vi "Add Measurement.vi"(8 "error in (no error)":errorcluster, 10 "Measurement":refnum<class "TestManagerMsg.Measurement.lvclass">, 11 "TestManagerMsg.Assertion in":refnum<class "TestManagerMsg.Assertion.lvclass">) -> (0 "error out":errorcluster, 1 "Created/Updated":bool, 3 "TestManagerMsg.Assertion out":refnum<class "TestManagerMsg.Assertion.lvclass">)   [LabVIEW 2013, in "Caraya.lvlib" / "TestManagerMsg.Assertion.lvclass"]
uses:
  TestManagerMsg.Assertion.lvclass
  Test Manager Message Measurement/TestManagerMsg.Measurement.lvclass
  TestManagerMsg.Assertion.lvclass/TestManagerMsg.Assertion.ctl
  Test Manager Message/TestManagerMsg.lvclass/TestManagerMsg.ctl
  Test Manager Message/TestManagerMsg.lvclass
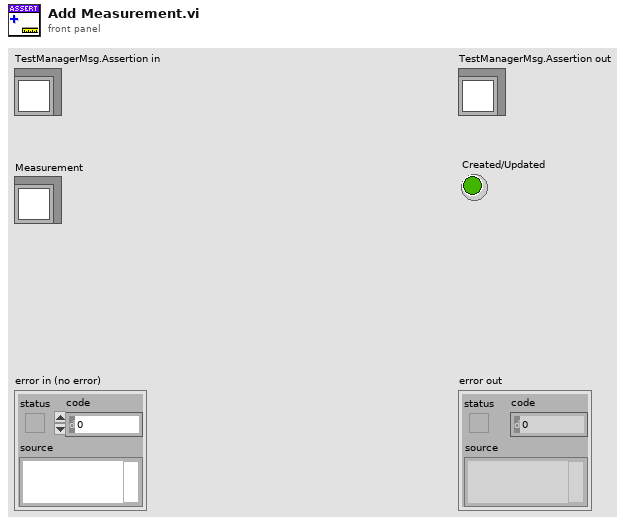
[diagram p1: front panel]
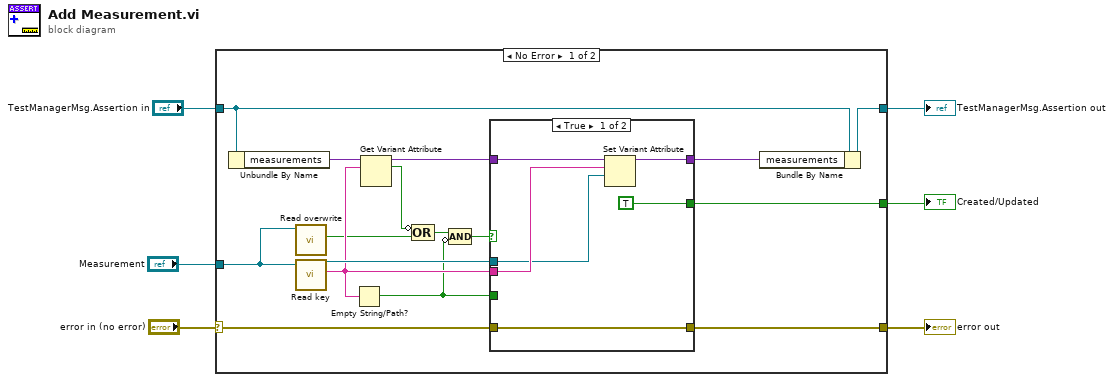
[diagram p0: block diagram]
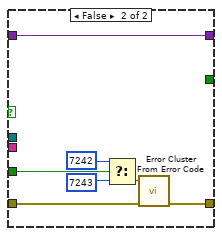
[diagram p2: hidden frame]
diagram:
  n1 = case shown="No Error" "error in (no error)" {
    selector: "error in (no error)" -> [w9 w37]
    tunnel: [w8 w37] -> w1
    tunnel: [w19 w36] -> w5
    tunnel: "TestManagerMsg.Assertion in" -> [w20 w36]
    tunnel: "Measurement" -> [w22 _]
    tunnel: [w10 _] -> w4
    frame No Error {
      n2 = Unbundle By Name(w20) -> ("measurements"=w17:variant)
      n3 = call "Read overwrite.vi"("TestManagerMsg in"=w22) -> ("overwrite?"=w14:bool)  [unwired: 9 in, 1 out]
      n4 = call "Read key.vi"("TestManagerMsg in"=w22) -> ("key"=w15:string, "TestManagerMsg out"=w18:refnum<class "TestManagerMsg.Measurement.lvclass">)  [unwired: 9 in]
      n5 = Empty String/Path?(string/path=w15) -> (empty?=w7:bool)
      n6 = Get Variant Attribute(Variant=w17, name=w15) -> (duplicate Variant=w16:variant, found=w13:bool)  [unwired: 2 in, 2 out]
      n7 = Compound Arithmetic op=OR(invert w13, w14) -> (w12:bool)
      n8 = Compound Arithmetic op=AND(w12, invert w7) -> (w11:bool)
      n9 = case shown="True" w11 {
        tunnel: w16 -> [w28 w35]
        tunnel: [w27 w35] -> w21
        tunnel: w15 -> [w26 _]
        tunnel: w18 -> [w25 _]
        tunnel: [TRUE _] -> w10
        tunnel: [w23 w34] -> w8
        tunnel: w9 -> [w23 w33]
        tunnel: w7 -> [_ w32]
        frame True {
          n10 = Set Variant Attribute(Variant=w28, name=w26, value=w25) -> (Variant out=w27:variant)  [unwired: 1 in, 2 out]
        }
        frame False {
          n11 = Select(t=7242 ("error code (0)"), s=w32, f=7243 ("error code (0)")) -> (s? t:f=w30:i32)
          n12 = call <vilib>:"Error Cluster From Error Code.vi"("error in (no error)"=w33, "error code (0)"=w30) -> ("error out"=w34:errorcluster)  [unwired: 7 in]
        }
      }
      n13 = Bundle By Name(cluster=w20, "measurements"=w21) -> (w19:refnum<class "TestManagerMsg.Assertion.lvclass">)
    }
    frame Error {
    }
  }
  "TestManagerMsg.Assertion out" <- w5
  "Created/Updated" <- w4
  "error out" <- w1
